vi "Pause.vi"(8 "error in":errorcluster, 9 "timeout (-1)":i32=-1, 11 "Standard Engine Runtime in":refnum<class "Standard Engine Runtime.lvclass">) -> (0 "error out":errorcluster, 3 "Standard Engine Runtime out":refnum<class "Standard Engine Runtime.lvclass">)   [LabVIEW 2013, in "Standard Engine Runtime.lvclass"]
doc: "This method will pause the execution of an engine in a running state. Call the 'Start' method to resume execution, or the 'Stop' method to have the engine shutdown."
uses:
  Standard Engine Runtime.lvclass
  engine state.ctl
  Standard Engine Runtime.lvclass/Standard Engine Runtime.ctl
  main engine/main engine.lvlib
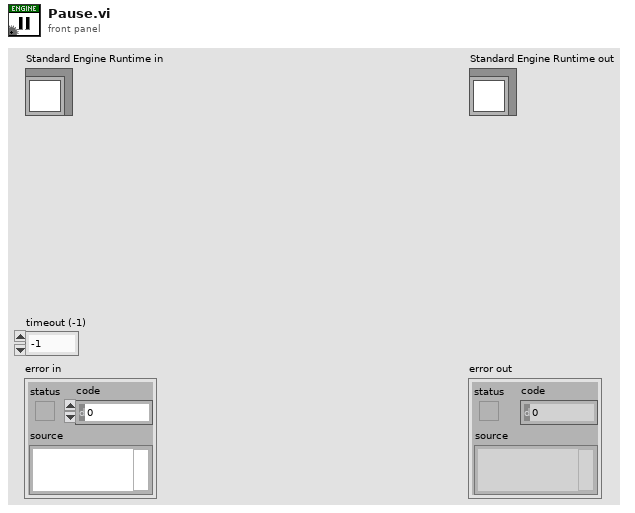
[diagram p1: front panel]
types:
  T1 = typedef "main engine.lvlib/engine state.ctl" = enum16{"idle", "configured", "running", "safe state", "exit"}
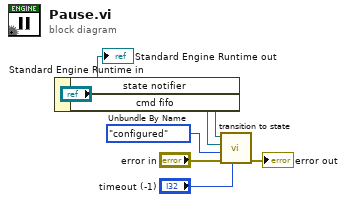
[diagram p0: block diagram]
diagram:
  n1 = Unbundle By Name("Standard Engine Runtime in") -> ("state notifier"=w3:refnum<notifier>, "cmd fifo"=w2:refnum<k33>)
  n2 = call "transition to state.vi"("timeout"="timeout (-1)", "error in"="error in", "state"=engine_state."configured" ("element"), "cmd fifo"=w2, "notifier"=w3) -> ("error out"=→"error out":errorcluster)  [unwired: 6 in]
  "Standard Engine Runtime out" <- "Standard Engine Runtime in"
